vi "V50 Report Fabric (SubVI).vi"(0 "NI_report in":refnum<class "NI_report.lvclass">, 5 "SampleID":string, 11 "error in (no error)":errorcluster) -> (4 "NI_report out":refnum<class "NI_report.lvclass">, 15 "error out":errorcluster)   [LabVIEW 2015]
uses:
  <vilib>/Utility/NIReport.llb/NI_report.lvclass
panel:
  out "appended array":string[][](array[string])
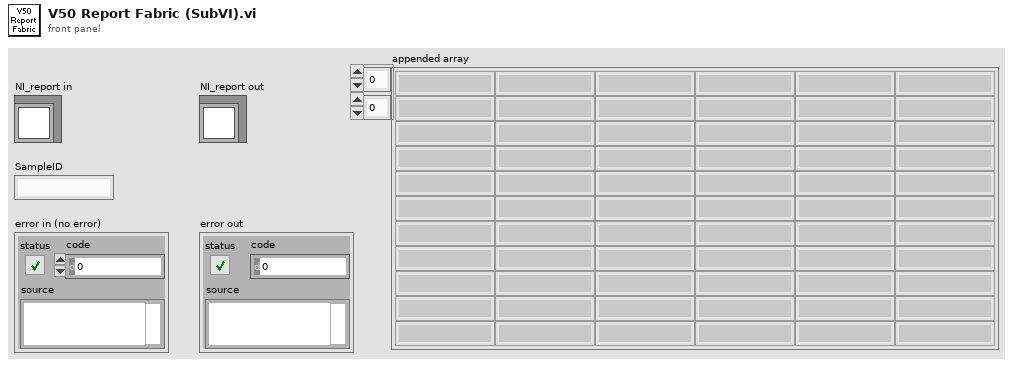
[diagram p1: front panel]
types:
  T1 = cluster{"position (excel)":cluster{"row":i32, "column":i32}, "name (excel)":string, "bookmark (word)":string}
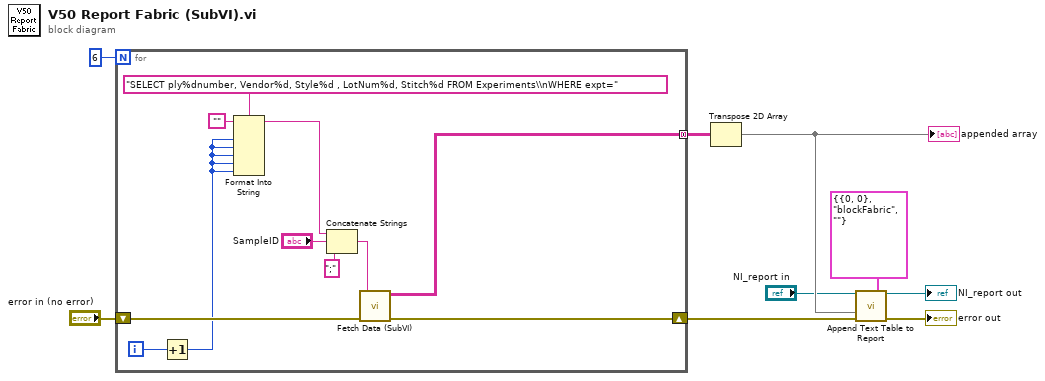
[diagram p0: block diagram]
diagram:
  n1 = for {
    N: 6 -> [_]
    tunnel: [w10] -> w6 mode=concatenating
    shift-right: [w16] -> w8
    shift-left: "error in (no error)" -> [w17]
    i -> [w12]
    n2 = Increment(x=w12) -> (x+1=w11:i32)
    n3 = Format Into String(format string="SELECT ply%dnumber, Vendor%d, Style%d , LotNum%d, Stitch%d FROM Experiments\\nWHERE expt=" ("query string"), initial string="", w11, w11, w11, w11, w11) -> (resulting string=w15:string)  [unwired: 1 in, 1 out]
    n4 = Concatenate Strings(w15, "SampleID", ";" ("string")) -> (w18:string)
    n5 = call "Fetch Data (SubVI).vi"("error IN"=w17, "query string"=w18) -> ("error OUT"=w16:errorcluster, "recordset data"=w10:string[][])  [unwired: 4 out]
  }
  n6 = Transpose 2D Array(2D array=w6) -> (transposed array=w5:string[][])
  "appended array" <- w5
  n7 = call-dynamic "Append Text Table to Report.vi"("report in"="NI_report in", "MS Office parameters"=T1 {"position (excel)"={"row"=0, "column"=0}, "name (excel)"="blockFabric", "bookmark (word)"=""}, "text data"=w5, "error in (no error)"=w8) -> ("report out"=→"NI_report out":refnum<class "NI_report.lvclass">, "error out"=→"error out":errorcluster)  [unwired: 8 in, 2 out]
